vi "Construct.vi"(8 "error in (no error)":errorcluster, 11 "CReporter in":refnum<class "CReporter.lvclass">) -> (0 "error out":errorcluster, 3 "CReporter out":refnum<class "CReporter.lvclass">)   [LabVIEW 2020, in "DependencyInspection.lvlib" / "CReporter.lvclass"]
uses:
  CReporter.lvclass
  CDependencyList/CDependencyList.lvclass
  CReporter.lvclass/CReporter.ctl
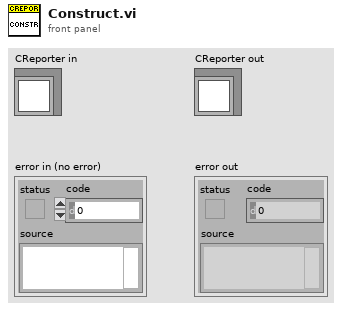
[diagram p1: front panel]
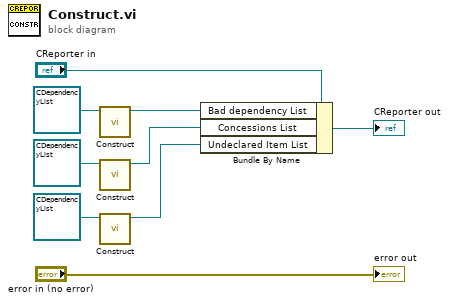
[diagram p0: block diagram]
diagram:
  n1 = call-dynamic "Construct.vi"("CDependencyList in"=refnum<class "CDependencyList.lvclass"> refnum ("Dependency List")) -> ("CDependencyList out"=w5:refnum<class "CDependencyList.lvclass">)  [unwired: 9 in, 1 out]
  n2 = call-dynamic "Construct.vi"("CDependencyList in"=refnum<class "CDependencyList.lvclass"> refnum ("Dependency List")) -> ("CDependencyList out"=w2:refnum<class "CDependencyList.lvclass">)  [unwired: 9 in, 1 out]
  n3 = call-dynamic "Construct.vi"("CDependencyList in"=refnum<class "CDependencyList.lvclass"> refnum ("Dependency List")) -> ("CDependencyList out"=w1:refnum<class "CDependencyList.lvclass">)  [unwired: 9 in, 1 out]
  n4 = Bundle By Name(cluster="CReporter in", "Bad dependency List"=w5, "Concessions List"=w2, "Undeclared Item List"=w1) -> (→"CReporter out":refnum<class "CReporter.lvclass">)
  "error out" <- "error in (no error)"
